vi "Read Config.vi"(8 "error in (no error)":errorcluster, 11 "FileName":string="SerialConfig.xml") -> (0 "error out":errorcluster, 3 "Serial Config":T1={"串口选择"="", "通讯速率"=9600, "超时时间"=10000, "数据位长"=8, "奇偶校验"=enum."None", "停止位长"=10, "握手控制"=0, "字符结束"=TRUE, "结束字符"=10, "仪器地址"=1} {"结束字符" format="%.0x"; "握手控制" items=["None", "XON/XOFF", "RTS/CTS", "XON/XOFF & RTS/CTS", "DTR/DSR", "XON/XOFF & DTR/DSR"]; "停止位长" items=["1.0"=10, "1.5"=15, "2.0"=20]; "数据位长" min=5 max=8 step=1})   [LabVIEW 2010, in "DCP551.lvlib"]
doc: "Use this template to build a VI to use as a subVI."
uses:
  DCP551.lvlib
  <vilib>/Utility/xml.llb/Read From XML File(string).vi
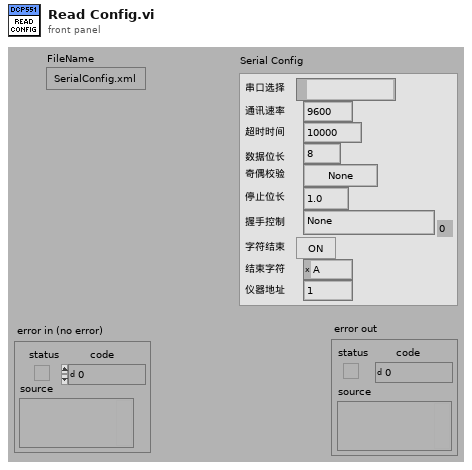
[diagram p1: front panel]
types:
  T1 = cluster{"串口选择":refnum<visa-resource-name>, "通讯速率":u32, "超时时间":u32, "数据位长":u16, "奇偶校验":enum16{"None", "Odd", "Even", "Mark", "Space"}, "停止位长":u16, "握手控制":u16, "字符结束":bool, "结束字符":u8, "仪器地址":u32}
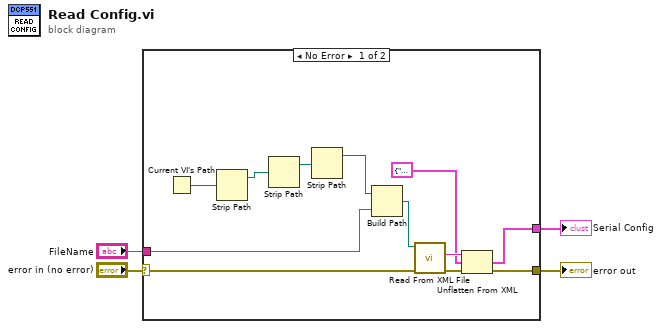
[diagram p0: block diagram]
diagram:
  n1 = case shown="No Error" "error in (no error)" {
    selector: "error in (no error)" -> [w13 w17]
    tunnel: [w11 w17] -> w3
    tunnel: "FileName" -> [w9 _]
    tunnel: [w8 _] -> w1
    frame No Error {
      n2 = Current VI's Path() -> (path=w15:path)
      n3 = Strip Path(path=w15) -> (stripped path=w6:path)  [unwired: 1 out]
      n4 = Strip Path(path=w6) -> (stripped path=w7:path)  [unwired: 1 out]
      n5 = Strip Path(path=w7) -> (stripped path=w5:path)  [unwired: 1 out]
      n6 = Build Path(base path=w5, name or relative path=w9) -> (appended path=w16:path)
      n7 = call-poly <vilib>:"Read From XML File.vi"("error in (no error)"=w13, "XML File Path"=w16) -> ("error out"=w12:errorcluster, "XML Elements"=w14:string)  [unwired: 7 in, 1 out]
      n8 = Unflatten From XML(xml string=w14, type=T1 {"串口选择"="COM1", "通讯速率"=9600, "超时时间"=10000, "数据位长"=8, "奇偶校验"=enum."None", "停止位长"=10, "握手控制"=0, "字符结束"=TRUE, "结束字符"=10, "仪器地址"=1} ("Serial Config 2"), error in (no error)=w12) -> (value=w8:T1, error out=w11:errorcluster)
    }
    frame Error {
    }
  }
  "error out" <- w3
  "Serial Config" <- w1
